vi "脉冲精度.vi"(10 "检验开始":bool, 11 "串口号":refnum<visa-resource-name>) -> (8 "应答":string)   [LabVIEW 2014]
panel:
  out "完整帧":u8[](array[numeric]) format="%.0x"
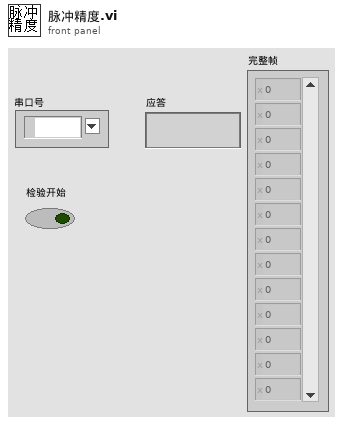
[diagram p1: front panel]
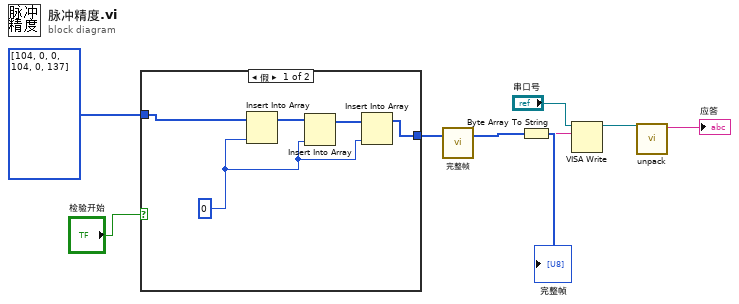
[diagram p0: block diagram]
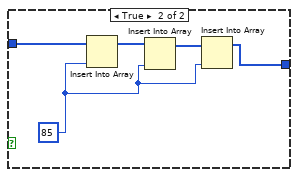
[diagram p2: hidden frame]
diagram:
  n1 = case shown="假" "检验开始" {
    tunnel: u8[] [104, 0, 0, 104, 0, 137] -> [w10 w15]
    tunnel: [w9 w14] -> w1
    frame False {
      w13 = 0
      n2 = Insert Into Array(array=w10, new element=w13) -> (w12:u8[])  [unwired: 1 in]
      n3 = Insert Into Array(array=w12, new element=w13) -> (w11:u8[])  [unwired: 1 in]
      n4 = Insert Into Array(array=w11, new element=w13) -> (w9:u8[])  [unwired: 1 in]
    }
    frame True {
      w18 = 85
      n5 = Insert Into Array(array=w15, new element=w18) -> (w17:u8[])  [unwired: 1 in]
      n6 = Insert Into Array(array=w17, new element=w18) -> (w16:u8[])  [unwired: 1 in]
      n7 = Insert Into Array(array=w16, new element=w18) -> (w14:u8[])  [unwired: 1 in]
    }
  }
  n8 = call "完整帧.vi"("不完整帧"=w1) -> ("完整帧"=w6:u8[])  [unwired: 2 in]
  "完整帧" <- w6
  n9 = Byte Array To String(unsigned byte array=w6) -> (string=w5:string)
  n10 = VISA Write(VISA resource name="串口号", write buffer=w5) -> (VISA resource name out=w3:refnum<visa-resource-name>)  [unwired: 1 in, 2 out]
  n11 = call "unpack.vi"("串口号输入"=w3) -> ("应答"=→"应答":string)  [unwired: 5 in, 1 out]
